vi "Plot.vi"(11 "Grid in":refnum<class "Grid.lvclass">) -> ()   [LabVIEW 2013, in "Grid.lvclass"]
uses:
  Grid.lvclass
  Controls/Neuron Info.ctl
  Controls/Type of Neuron.ctl
  Grid.lvclass/Grid.ctl
  <vilib>/Utility/miscctls.llb/LV3DPointTypeDef.ctl
  <vilib>/Analysis/coordinate.llb/3D Coordinate Conversion (Scalar).vi
  <vilib>/Analysis/NI_AALPro.lvlib
panel:
  out "Neurons Info":T1
  out "No Neurons":i32
  in  "stop":bool
  in  "Camera Position":cluster{"X":sgl, "Y":sgl, "Z":sgl}={"X"=0.0, "Y"=250.0, "Z"=100.0}
  out "3D Picture":refnum<vi>(3d-picture)
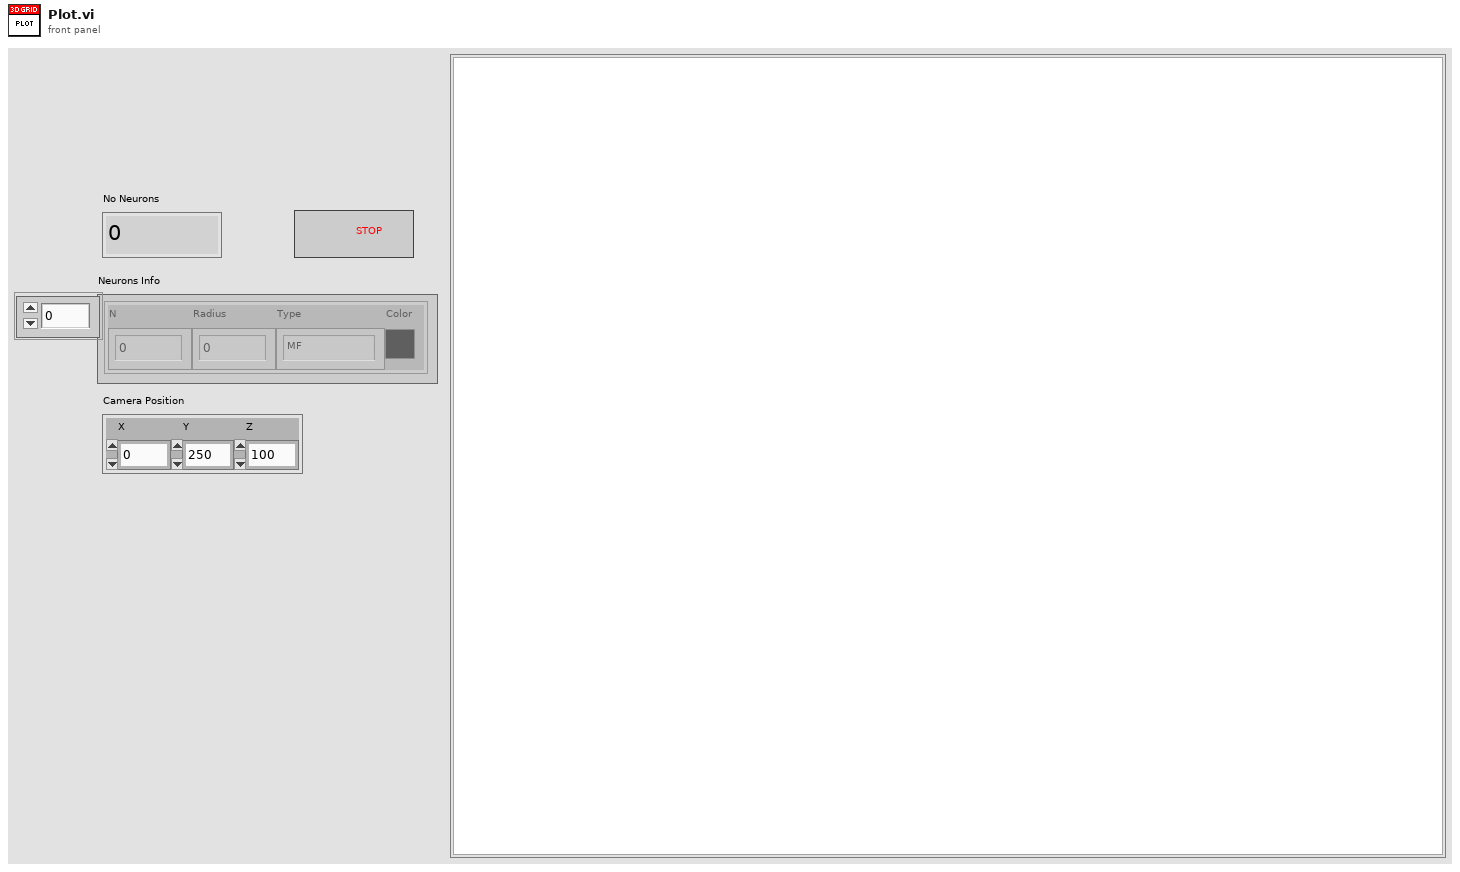
[diagram p1: front panel]
types:
  T1 = typedef "Neuron Info.ctl" = cluster{"N":i32, "Radius":dbl, "Type":T2, "Color":u32}[]
  T2 = typedef "Type of Neuron.ctl" = enum16{"MF", "BA", "GO", "GC", "PC", "LU", "Glia (Dummy)"}
  T3 = typedef "LV3DPointTypeDef.ctl" = cluster{"X":sgl, "Y":sgl, "Z":sgl}
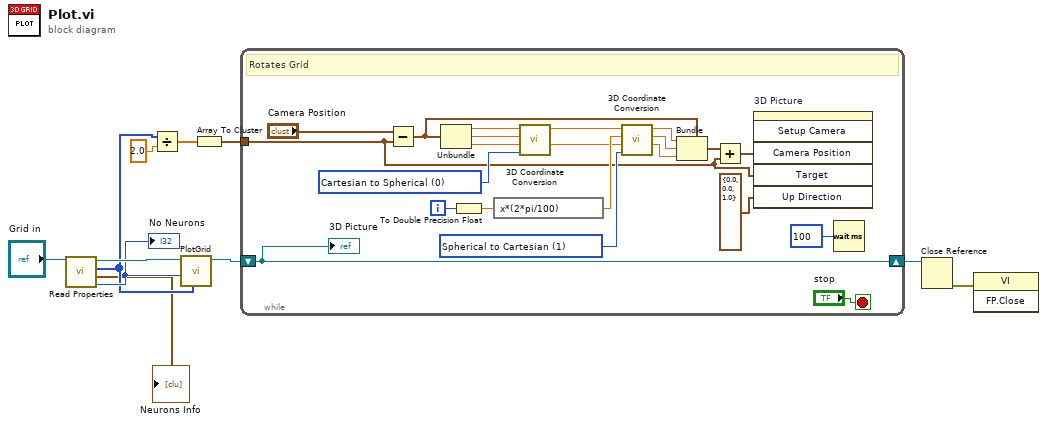
[diagram p0: block diagram]
diagram:
  n1 = call "Read Properties.vi"("Grid in"="Grid in") -> ("No Neurons"=w8:i32, "Neurons Info"=→"Neurons Info":T1, "Size(um)"=w5:u32[], "Grid out"=w9:refnum<class "Grid.lvclass">)  [unwired: 6 in, 1 out]
  "No Neurons" <- w8
  n2 = Divide(x=w5, y=2.0 ("Numeric")) -> (x/y=w6:dbl[])
  n3 = call "PlotGrid.vi"("Size (um)"=w5, "No Neurons"=w8, "Grid in"=w9) -> ("Scene Object Out"=w10:refnum<vi>)  [unwired: 8 in]
  n4 = Array To Cluster(array=w6) -> (cluster=w4:cluster{"[0]":dbl, "[1]":dbl, "[2]":dbl})
  n5 = while {
    shift-right: [w33] -> w11
    shift-left: w10 -> [w33]
    tunnel: w4 -> [w12]
    i -> [w28]
    stop <- "stop" stop-if-true
    w25 = u16 1 items=["Cartesian to Spherical", "Spherical to Cartesian", "Cartesian to Cylindrical", "Cylindrical to Cartesian", "Spherical to Cylindrical", "Cylindrical to Spherical"] ("conversion type")
    w29 = u16 0 items=["Cartesian to Spherical", "Spherical to Cartesian", "Cartesian to Cylindrical", "Cylindrical to Cartesian", "Spherical to Cylindrical", "Cylindrical to Spherical"] ("conversion type")
    # "Rotates Grid"
    n6 = Subtract(x="Camera Position", y=w12) -> (x-y=w15:cluster{dbl, dbl, dbl})
    n7 = Unbundle(w15) -> (w32:dbl, w31:dbl, w30:dbl)
    n8 = To Double Precision Float(number=w28) -> (double precision float=w27:dbl)
    n9 = expression code="x*(2*pi/100)"(w27) -> (w18:dbl)
    n10 = call-poly <vilib>:"3D Coordinate Conversion.vi"("conversion type"=w29, "axis 3"=w30, "axis 2"=w31, "axis 1"=w32) -> ("axis 3 out"=w17:dbl, "axis 1 out"=w26:dbl)  [unwired: 4 in, 2 out]
    n11 = call-poly <vilib>:"3D Coordinate Conversion.vi"("conversion type"=w25, "axis 3"=w17, "axis 2"=w18, "axis 1"=w26) -> ("axis 3 out"=w22:dbl, "axis 2 out"=w23:dbl, "axis 1 out"=w24:dbl)  [unwired: 4 in, 1 out]
    n12 = Bundle(cluster=w15, w24, w23, w22) -> (w14:cluster{dbl, dbl, dbl})
    n13 = Add(x=w14, y=w12) -> (x+y=w13:cluster{dbl, dbl, dbl})
    n14 = invoke on="3D Picture" class="SceneGraphDisp (strict)" method="Setup Camera"("Camera Position"=w13, "Target"=w12, "Up Direction"=T3 {"X"=0.0, "Y"=0.0, "Z"=1.0}) -> ()  [unwired: 3 in, 6 out]
    n15 = Wait (ms)(milliseconds to wait=u32 100) -> ()  [unwired: 1 out]
    "3D Picture" <- w33
  }
  n16 = Close Reference(reference=w11) -> (error out=w3:errorcluster)  [unwired: 1 in]
  n17 = invoke class="VI" method="FP.Close"(error in=w3) -> ()  [unwired: 2 in, 3 out]
